vi "Create DAQmx.AO.vi"(8 "error in (no error)":errorcluster, 9 "DAQmx.AO.config":T1={"output terminal configuration"=-1} {"output terminal configuration" items=["Default"=-1, "RSE"=10083, "Differential"=10106, "Pseudodifferential"=12529]}, 10 "DAQ.Config":T2={"Channels"="", "DAQType"=enum."AI", "minimum value"=-5.0, "maximum value"=5.0, "sampling info"={"Fs"=1000.0, "#s"=1000.0}, "SamplingMode"=enum."Continuous"} {"maximum value" format="%0.2f"; "minimum value" format="%0.2f"}, 11 "DAQmx.AO in":refnum<class "DAQmx.AO.lvclass">) -> (0 "error out":errorcluster, 3 "DAQmx.AO out":refnum<class "DAQmx.AO.lvclass">)   [LabVIEW 2016, in "DAQmx.AO.lvclass"]
uses:
  DAQmx.AO.lvclass
  C:/user/patrick/hg/lockin.SMO/lvsrc/SMOs/DAQmx/DAQmx.lvclass
  DAQ/Typedefs/DAQ.Config.ctl
  DAQ/Typedefs/PrivateEvents--DAQ.AI.Channels.ctl
  DAQ/Typedefs/DAQType.ctl
  DAQ/Typedefs/SamplingInfo.ctl
  DAQ/Typedefs/SamplingMode.ctl
  Typedefs/DAQmx.AO.Config.ctl
  DAQmx.AO.lvclass/DAQmx.AO.ctl
  DAQmx/DAQmx.lvclass
  DAQ/DAQ.lvclass
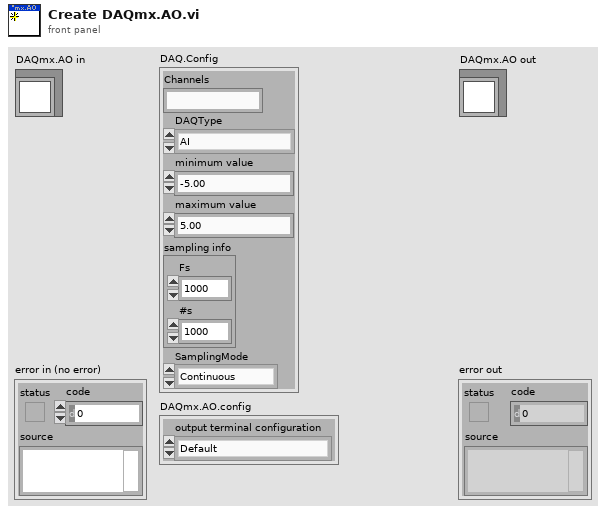
[diagram p1: front panel]
types:
  T1 = typedef "DAQmx.AO.lvclass/DAQmx.AO.Config.ctl" = cluster{"output terminal configuration":i32}
  T2 = typedef "DAQ.lvclass/DAQ.Config.ctl" = cluster{"Channels":T3, "DAQType":T4, "minimum value":dbl, "maximum value":dbl, "sampling info":T5, "SamplingMode":T6}
  T3 = typedef "DAQ.lvclass/PrivateEvents--DAQ.AI.Channels.ctl" = string
  T4 = typedef "DAQ.lvclass/DAQType.ctl" = enum16{"AI", "AO"}
  T5 = typedef "DAQ.lvclass/SamplingInfo.ctl" = cluster{"Fs":dbl, "#s":dbl}
  T6 = typedef "DAQ.lvclass/SamplingMode.ctl" = enum16{"Continuous", "Finite"}
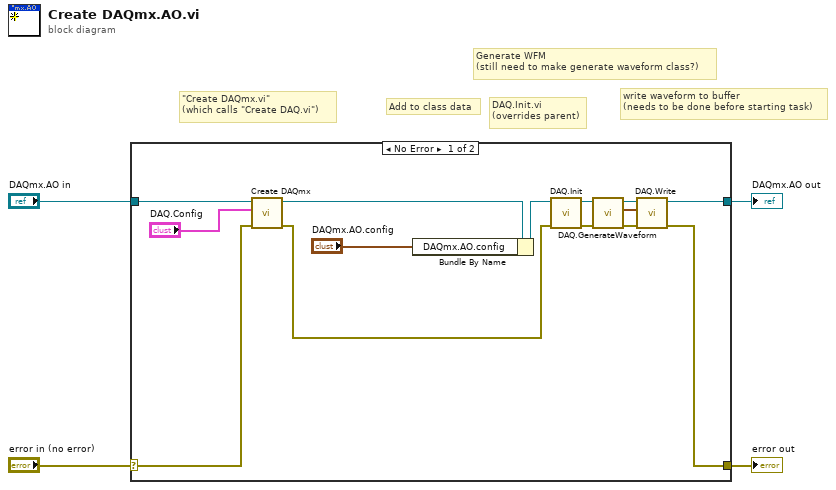
[diagram p0: block diagram]
diagram:
  # "write waveform to buffer\n(needs to be done before starting task)"
  # "Generate WFM\n(still need to make generate waveform class?)"
  # "\"Create DAQmx.vi\"\n(which calls \"Create DAQ.vi\")"
  # "Add to class data"
  # "DAQ.Init.vi\n(overrides parent)"
  n1 = case shown="No Error" "error in (no error)" {
    selector: "error in (no error)" -> [w15 w20]
    tunnel: [w11 w20] -> w3
    tunnel: [w10 w19] -> w1
    tunnel: "DAQmx.AO in" -> [w18 w19]
    frame No Error {
      n2 = call "Create DAQmx.vi"("error in (no error)"=w15, "DAQ.Config"="DAQ.Config", "DAQmx in"=w18) -> ("error out"=w12:errorcluster, "DAQmx out"=w14:refnum<class "DAQmx.AO.lvclass">)  [unwired: 7 in]
      n3 = Bundle By Name(cluster=w14, "DAQmx.AO.config"="DAQmx.AO.config") -> (w13:refnum<class "DAQmx.AO.lvclass">)
      n4 = call-dynamic "DAQ.Init.vi"("error in (no error)"=w12, "DAQmx.AO in"=w13) -> ("error out"=w5:errorcluster, "DAQmx.AO out"=w9:refnum<class "DAQmx.AO.lvclass">)  [unwired: 8 in]
      n5 = call-dynamic "DAQ.GenerateWaveform.vi"("error in (no error)"=w5, "DAQ in"=w9) -> ("error out"=w6:errorcluster, "Waveforms"=w7:waveform(dbl)[], "DAQ out"=w8:refnum<class "DAQmx.AO.lvclass">)  [unwired: 7 in]
      n6 = call-dynamic "DAQ.Write.vi"("error in (no error)"=w6, "Write"=w7, "DAQmx.AO in"=w8) -> ("error out"=w11:errorcluster, "DAQmx.AO out"=w10:refnum<class "DAQmx.AO.lvclass">)  [unwired: 7 in]
    }
    frame Error {
    }
  }
  "error out" <- w3
  "DAQmx.AO out" <- w1
